vi "Thread@Call__Parameter.vi"(1 "ParamterIn":string) -> (0 "ParamterOut":string)   [LabVIEW 2020]
panel:
  in  "Logic":string(combo)
  in  "Program":string(combo)="1"
  in  "Confirm":bool
  # "Thread@Call $Program(, $Logic)"
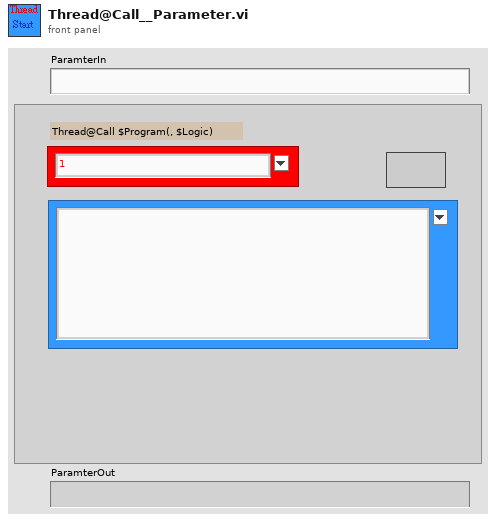
[diagram p1: front panel]
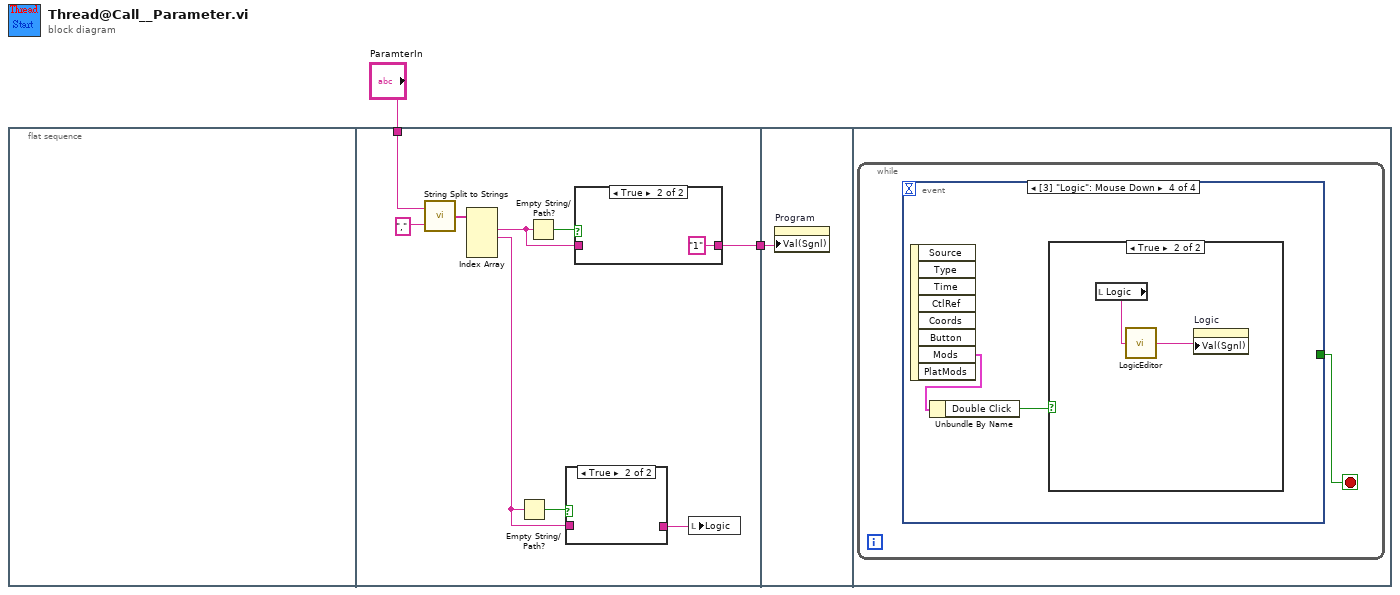
[diagram p0: block diagram]
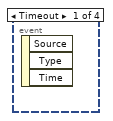
[diagram p4: hidden frame]
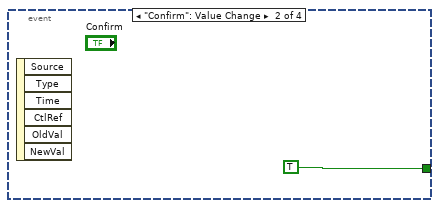
[diagram p5: hidden frame]
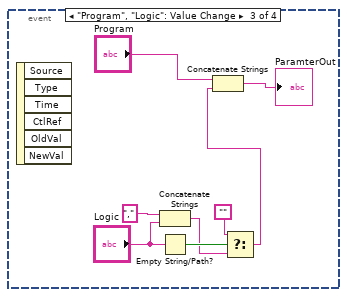
[diagram p6: hidden frame]
diagram:
  n1 = flat-sequence {
    tunnel: "ParamterIn" -> [w9]
    tunnel: [w6] -> w1
    tunnel: w1 -> [w15]
    frame #0 {
    }
    frame #1 {
      n2 = call "String Split to Strings.vi"("search string/char (-)"=",", "String"=w9) -> ("Array"=w11:string[])
      n3 = Index Array(array=w11) -> (element #1=w7:string, element #2=w3:string)  [unwired: 4 in, 2 out]
      n4 = Empty String/Path?(string/path=w3) -> (empty?=w5:bool)
      n5 = Empty String/Path?(string/path=w7) -> (empty?=w8:bool)
      n6 = case shown="True" w5 {
        tunnel: w3 -> [w12 _]
        tunnel: [w12 _] -> w4
        frame False {
        }
        frame True {
        }
      }
      n7 = case shown="True" w8 {
        tunnel: w7 -> [w13 _]
        tunnel: [w13 "1"] -> w6
        frame False {
        }
        frame True {
        }
      }
      n8 = local write "Logic"(w4) -> ()
    }
    frame #2 {
      n9 = property on="Program" class="CmbBox"("Val(Sgnl)"=w15) -> ()  [unwired: 2 in, 2 out]
    }
    frame #3 {
      n10 = while {
        stop <- w16 stop-if-true
        n11 = event shown="[3] \"Logic\": Mouse Down" {
          selector: _ -> [_ _ _ _]
          dyn-events: _ -> [_ _ _ _]
          timeout: _ -> [_ _ _ _]
          tunnel: [_ TRUE _ _] -> w16
          event Timeout {
            n12 = event-data() -> ()  [unwired: 1 in, 3 out]
          }
          event "Confirm": Value Change {
            n13 = event-data() -> ()  [unwired: 1 in, 6 out]
          }
          event "Program", "Logic": Value Change {
            n14 = event-data() -> ()  [unwired: 1 in, 6 out]
            n15 = Concatenate Strings("," ("string"), "Logic") -> (w20:string)
            n16 = Empty String/Path?(string/path="Logic") -> (empty?=w23:bool)
            n17 = Select(t="", s=w23, f=w20) -> (s? t:f=w18:string)
            n18 = Concatenate Strings("Program", w18) -> (→"ParamterOut":string)
          }
          event "Logic": Mouse Down {
            n19 = event-data() -> ("Mods"=w27:cluster{"Double Click":bool, "Menu Key":bool})  [unwired: 1 in, 7 out]
            n20 = Unbundle By Name(w27) -> ("Double Click"=w26:bool)
            n21 = case shown="True" w26 {
              frame False {
              }
              frame True {
                n22 = local read "Logic"() -> (w29:string)
                n23 = call "LogicEditor.vi"("Logic Express"=w29) -> ("LogicExpressOut"=w28:string)
                n24 = property on="Logic" class="CmbBox"("Val(Sgnl)"=w28) -> ()  [unwired: 2 in, 2 out]
              }
            }
          }
        }
      }
    }
  }
